vi "publish -- read -- num -- V2.vi"(8 "request event":refnum<user-event>) -> ()   [LabVIEW 2018]
panel:
  out "request event out":refnum<user-event>
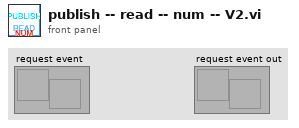
[diagram p1: front panel]
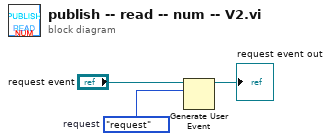
[diagram p0: block diagram]
diagram:
  w3 = enum16{"request"}."request"  # request
  n1 = Generate User Event(user event="request event", event data cluster=w3) -> (user event out=→"request event out":refnum<user-event>)  [unwired: 2 in, 1 out]
